vi "Count.vi"(8 "error in (no error)":errorcluster, 10 "计时":dbl=12.0 format="%0.8f", 11 "Time in":refnum<class "Time.lvclass">) -> (0 "error out":errorcluster, 1 "Time has Elapsed":bool, 2 "倒计时":dbl, 3 "Time out":refnum<class "Time.lvclass">)   [LabVIEW 2015, in "Time.lvclass"]
uses:
  Time.lvclass
  Time.lvclass/Time.ctl
panel:
  out "Elapsed Time":dbl format="%0.2f"
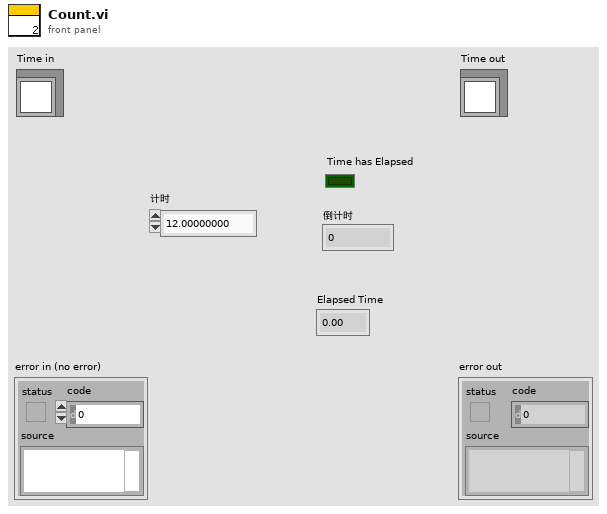
[diagram p1: front panel]
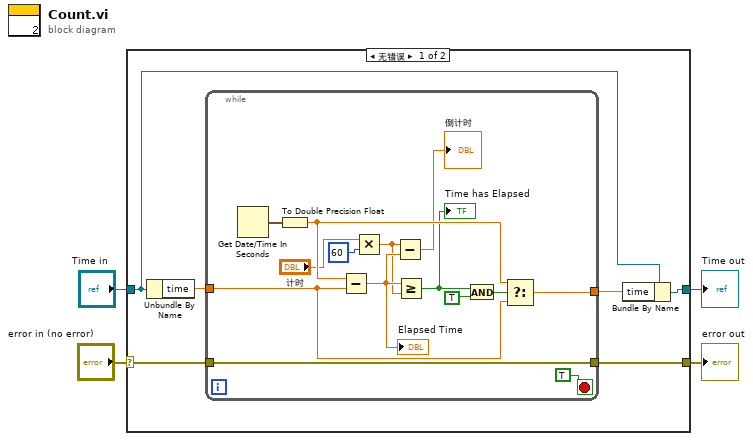
[diagram p0: block diagram]
diagram:
  n1 = case shown="无错误" "error in (no error)" {
    selector: "error in (no error)" -> [w9 w26]
    tunnel: [w8 w26] -> w3
    tunnel: [w5 w25] -> w1
    tunnel: "Time in" -> [w7 w25]
    frame No Error {
      n2 = Unbundle By Name(w7) -> ("time"=w10:dbl)
      n3 = while {
        tunnel: w10 -> [w12]
        tunnel: [w13] -> w6
        tunnel: w9 -> [w11]
        tunnel: [w11] -> w8
        stop <- TRUE stop-if-true
        n4 = Get Date/Time In Seconds() -> (seconds since 1Jan1904=w21:timestamp)
        n5 = To Double Precision Float(number=w21) -> (double precision float=w20:dbl)
        n6 = Subtract(x=w20, y=w12) -> (x-y=w19:dbl)
        "Elapsed Time" <- w19
        n7 = Multiply(x="计时", y=60) -> (x*y=w15:dbl)
        n8 = Subtract(x=w15, y=w19) -> (x-y=→"倒计时":dbl)
        n9 = Greater Or Equal?(x=w19, y=w15) -> (x >= y?=w18:bool)
        "Time has Elapsed" <- w18
        n10 = And(x=w18, y=TRUE ("Auto Reset")) -> (x .and. y?=w22:bool)
        n11 = Select(t=w20, s=w22, f=w12) -> (s? t:f=w13:dbl)
      }
      n12 = Bundle By Name(cluster=w7, "time"=w6) -> (w5:refnum<class "Time.lvclass">)
    }
    frame Error {
    }
  }
  "error out" <- w3
  "Time out" <- w1
